vi "DepthSense Global Status.vi"() -> ()   [LabVIEW 2011]
uses:
  DepthSense State.ctl
  <vilib>/vision/Image Controls.llb/IMAQ Image.ctl
panel:
  in  "Try Me":dbl
  in  "Depth Image Queue":refnum<queue>
  in  "DepthSense Status":T1={"Camera Version"="", "Image Height"=0, "Image Width"=0, "Minimum Framerate"=0, "Maximum Framerate"=0, "Framerate"=25, "Close Mode"=FALSE, "Denoising"=TRUE, "Leakage Algorithm"=TRUE, "Anti-Aliasing"=TRUE, "Camera Status"=-2, "API Version"="", "Light Intensity"=100}
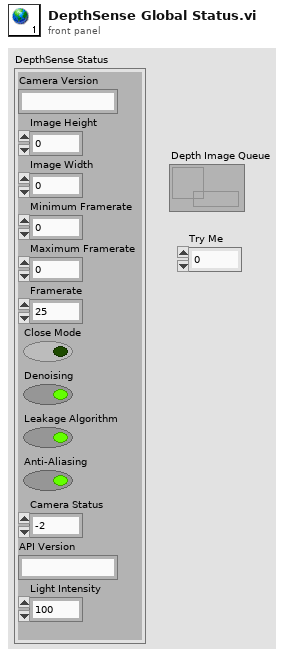
[diagram p1: front panel]
types:
  T1 = typedef "DepthSense State.ctl" = cluster{"Camera Version":string, "Image Height":i32, "Image Width":i32, "Minimum Framerate":i32, "Maximum Framerate":i32, "Framerate":i32, "Close Mode":bool, "Denoising":bool, "Leakage Algorithm":bool, "Anti-Aliasing":bool, "Camera Status":i32, "API Version":string, "Light Intensity":i32}
diagram:
